vi "Monitor Current Position.vi"(8 "error in (no error)":errorcluster, 9 "Y-Axis In":refnum<class "iMotion Controller.lvclass">, 10 "X-Axis In":refnum<class "iMotion Controller.lvclass">, 11 "Stage Data Class":refnum<data-value>) -> (0 "error out":errorcluster, 1 "Y-Axis Out":refnum<class "iMotion Controller.lvclass">, 2 "X-Axis Out":refnum<class "iMotion Controller.lvclass">, 3 "Stage Data Class":refnum<data-value>)   [LabVIEW 2022 SP3, in "XY Stage Process.lvlib" / "XY Stage Process.lvclass"]
uses:
  XY Stage Process.lvclass
  XY Stage Process.lvclass/XY Stage Process.ctl
  6046c730-44da-4461-abcf-74f1f8a9aa6a.vi
  Axis Objects/iMotion Controller/iMotion Controller.lvclass
  XY Stage Data Class/XY Position.ctl
  XY Stage Data Class/XY Stage Data Class.lvclass
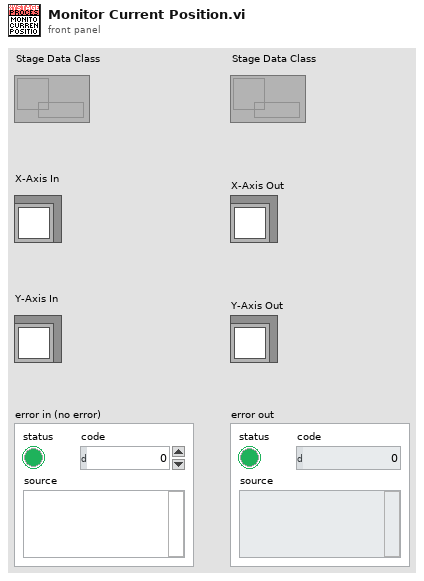
[diagram p1: front panel]
types:
  T1 = typedef "XY Stage Data Class.lvclass/XY Position.ctl" = cluster{"Current Position X":dbl, "Current Position Y":dbl}
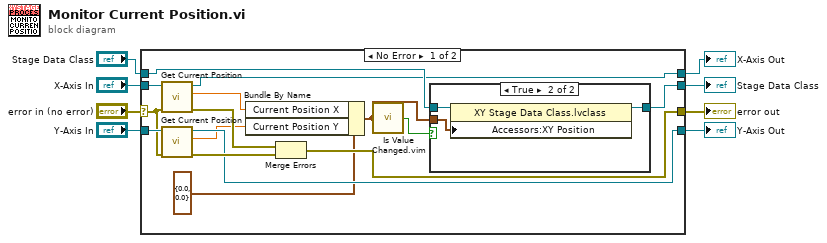
[diagram p0: block diagram]
diagram:
  n1 = case shown="No Error" "error in (no error)" {
    selector: "error in (no error)" -> [w19 w28]
    tunnel: "Y-Axis In" -> [w22 w29]
    tunnel: "X-Axis In" -> [w21 w30]
    tunnel: "Stage Data Class" -> [w20 w31]
    tunnel: [w16 w31] -> w4
    tunnel: [w15 w30] -> w3
    tunnel: [w14 w29] -> w2
    tunnel: [w13 w28] -> w1
    frame No Error {
      n2 = call-dynamic "Get Current Position.vi"("error in (no error)"=w19, "iMotion Controller in"=w21) -> ("error out"=w18:errorcluster, "Current Position"=w11:dbl, "iMotion Controller out"=w15:refnum<class "iMotion Controller.lvclass">)  [unwired: 7 in]
      n3 = call-dynamic "Get Current Position.vi"("error in (no error)"=w19, "iMotion Controller in"=w22) -> ("error out"=w17:errorcluster, "Current Position"=w10:dbl, "iMotion Controller out"=w14:refnum<class "iMotion Controller.lvclass">)  [unwired: 7 in]
      n4 = Bundle By Name(cluster=T1 {"Current Position X"=0.0, "Current Position Y"=0.0} ("XY Position"), "Current Position X"=w11, "Current Position Y"=w10) -> (w9:T1)
      n5 = Merge Errors(w18, w17) -> (w13:errorcluster)
      n6 = call "Is Value Changed.vim"("value"=w9) -> ("changed or first call?"=w23:bool)
      n7 = case shown="True" w23 {
        tunnel: [w24 w27] -> w16
        tunnel: w20 -> [w24 w26]
        tunnel: w9 -> [_ w25]
        frame False {
        }
        frame True {
          n8 = property class="XY Stage Data Class.lvclass"(reference=w26, "Accessors:XY Position"=w25) -> (reference out=w27:refnum<data-value>)  [unwired: 1 in, 1 out]
        }
      }
    }
    frame Error {
    }
  }
  "Stage Data Class" <- w4
  "X-Axis Out" <- w3
  "Y-Axis Out" <- w2
  "error out" <- w1
